vi "Autonomous Tipping.vi"() -> ()   [LabVIEW 2012]
panel:
  in  "Autonomous Tipping":bool
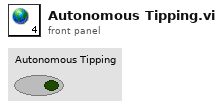
[diagram p1: front panel]
diagram:
